vi "Generate Tabs.vi"(8 "error in (no error)":errorcluster) -> (0 "error out":errorcluster, 2 "Tabs":string)   [LabVIEW 2015, in "LVJSON.lvlib"]
uses:
  LVJSON.lvlib
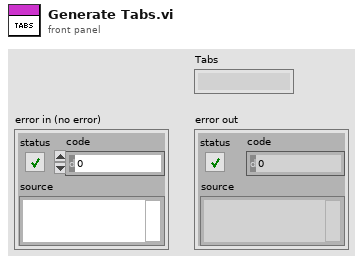
[diagram p1: front panel]
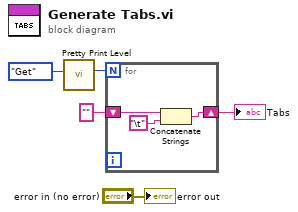
[diagram p0: block diagram]
diagram:
  n1 = call "Pretty Print Level.vi"("Action"=enum16{"Increment", "Decrement", "Get", "Reset"}."Get") -> ("Numeric"=w4:i32)  [unwired: 9 in, 1 out]
  n2 = for {
    N: w4 -> [_]
    shift-right: [w6] -> w2
    shift-left: "" -> [w8]
    n3 = Concatenate Strings(w8, "\t") -> (w6:string)
  }
  "Tabs" <- w2
  "error out" <- "error in (no error)"
